vi "inputView.vi"(10 "UserEvents in":refnum<class "UserEvents.lvclass">) -> ()   [LabVIEW 2015, in "M1M3SSSTViews.lvlib"]
uses:
  M1M3SSSTViews.lvlib
  UserEvents/UserEvents.lvclass
  UserEvents/UserEvents.lvclass/UserEvents.ctl
  Typedefs/StateSelector.ctl
  Typedefs/M1M3SSSTypedefs.lvlib
panel:
  out "Distance Measured":dbl[unit]=25399.999999999996 min=25399.999999999996 max=7620000.0 format="%.3f"
  out "Force Measured":dbl[unit] min=-888.0 max=888.0 format="%.2f"
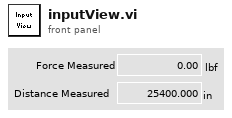
[diagram p1: front panel]
types:
  T1 = typedef "M1M3SSSTypedefs.lvlib/PubDataEvents.ctl" = cluster{"State":refnum<user-event>, "ErrorCode":refnum<user-event>, "OutputData":refnum<user-event>, "InputData":refnum<user-event>, "ControllerData":refnum<user-event>, "TestStatus":refnum<user-event>, "LogPath":refnum<user-event>, "StiffnessData":refnum<user-event>, "PreconditioningCycle":refnum<user-event>}
  T2 = cluster{"Event Registration Refnum":refnum<event-registration>, "Event Registration Refnum":refnum<event-registration>}
  T3 = typedef "M1M3SSSTypedefs.lvlib/StateSelector.ctl" = enum16{"FaultState", "OffState", "RampingUpPressurePState", "RampingUpPressureSTState", "StandbyState", "StoppedState", "WaitingForSettledPState", "WaitingForSettledSTState"}
  T4 = typedef "M1M3SSSTypedefs.lvlib/ForceDemand.ctl" = dbl[unit]
  T5 = typedef "DistanceGauge.lvlib/Distance Data.ctl" = cluster{"Distance Measured":dbl[unit]}
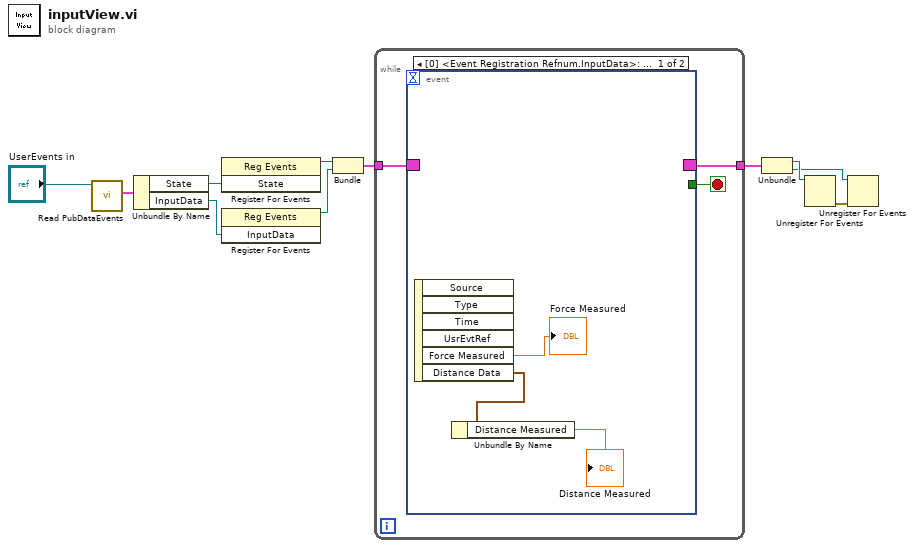
[diagram p0: block diagram]
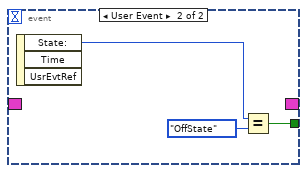
[diagram p2: hidden frame]
diagram:
  n1 = call "Read PubDataEvents.vi"("UserEvents in"="UserEvents in") -> ("PubDataEvents"=w11:T1)  [unwired: 9 in, 1 out]
  n2 = Unbundle By Name(w11) -> ("State"=w10:refnum<user-event>, "InputData"=w8:refnum<user-event>)
  n3 = register-events(w10) -> (reference out=w9:refnum<event-registration>)  [unwired: 2 in, 1 out]
  n4 = register-events(w8) -> (reference out=w7:refnum<event-registration>)  [unwired: 2 in, 1 out]
  n5 = Bundle("Event Registration Refnum"=w9, "Event Registration Refnum"=w7) -> (w5:T2)  [unwired: 1 in]
  n6 = while {
    tunnel: w5 -> [w14]
    tunnel: [w12] -> w4
    stop <- w13 stop-if-true
    n7 = event shown="[0] <Event Registration Refnum.InputData>: User Event" {
      selector: w14 -> [_ _]
      dyn-events: [_ _] -> w12
      timeout: _ -> [_ _]
      tunnel: [_ w19] -> w13
      event User Event {
        n8 = event-data() -> ("Force Measured"=→"Force Measured":T4, "Distance Data"=w15:T5)  [unwired: 1 in, 4 out]
        n9 = Unbundle By Name(w15) -> ("Distance Measured"=→"Distance Measured":dbl[unit])
      }
      event User Event {
        n10 = event-data() -> ("State:"=w18:T3)  [unwired: 1 in, 2 out]
        n11 = Equal?(x=w18, y=StateSelector."OffState" ("State:")) -> (x = y?=w19:bool)
      }
    }
  }
  n12 = Unbundle(w4) -> ("Event Registration Refnum"=w3:refnum<event-registration>, "Event Registration Refnum"=w2:refnum<event-registration>)
  n13 = Unregister For Events(event registration refnum=w3) -> (error out=w1:errorcluster)  [unwired: 1 in]
  n14 = Unregister For Events(event registration refnum=w2, error in=w1) -> ()  [unwired: 1 out]
